vi "The Red LED.vi"() -> ()   [LabVIEW 2020]
uses:
  Red Button Enum.ctl
panel:
  out "error out":errorcluster
  in  "Open time duration(s)":u32=3
  in  "Switch":bool
  out "State":T1
  in  "stop":bool
  in  "1":bool
  in  "2":bool
  in  "3":bool
  out "Lamp":bool
  in  "Check for every step":bool
  # "The password is \"1-2-3\" consequtively, you should push \"check for every step\" in each step\nafter you select the number,  then switch and red LED indicator will be enabled. So as last step turn on the switch, LED will be open for 3 secs by default. You can easily change the password by giving desired boolean values inside case structure in the 1,2,3 cases, in the block diagram."
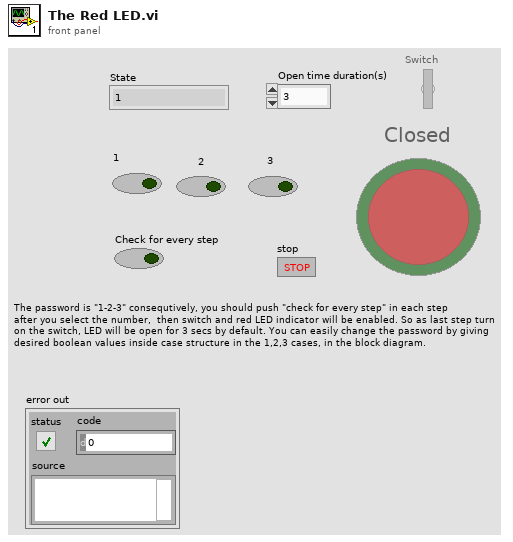
[diagram p1: front panel]
types:
  T1 = typedef "Red Button Enum.ctl" = enum16{"1", "2", "3", "Unlocked", "Open"}
  T2 = enum8{"Enabled", "Disabled", "Disabled and Grayed Out"}
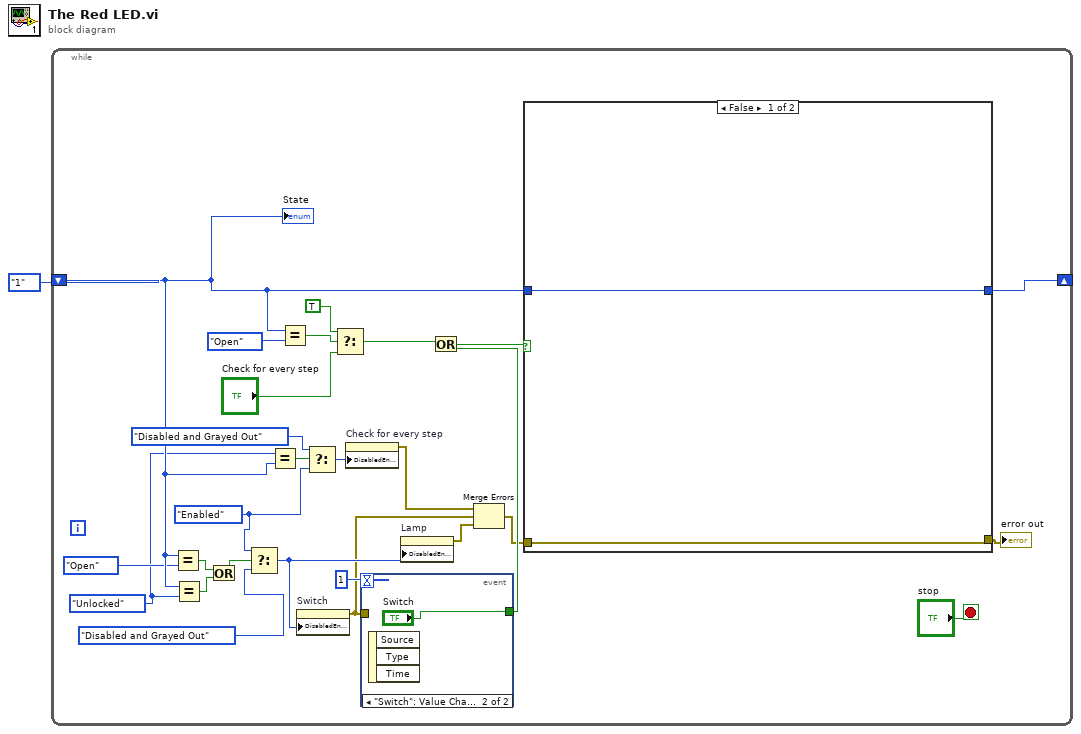
[diagram p0: block diagram]
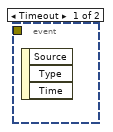
[diagram p2: hidden frame]
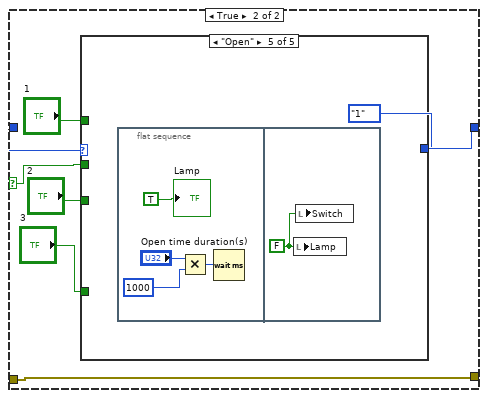
[diagram p3: hidden frame]
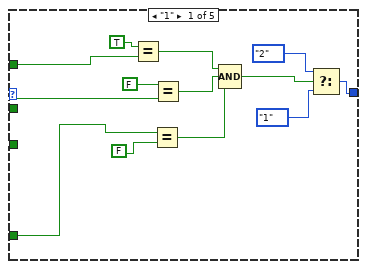
[diagram p4: hidden frame]
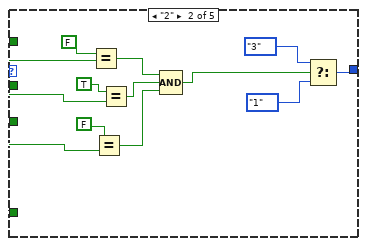
[diagram p5: hidden frame]
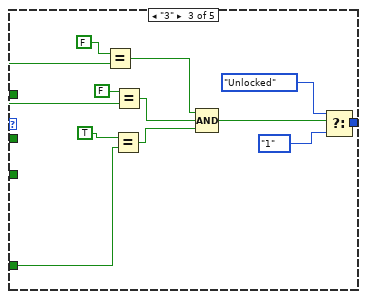
[diagram p6: hidden frame]
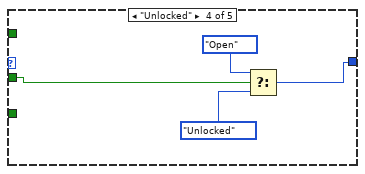
[diagram p7: hidden frame]
diagram:
  n1 = while {
    shift-right: [w27] -> _
    shift-left: Red_Button_Enum."1" ("Enum") -> [w13]
    stop <- "stop" stop-if-true
    w9 = T2."Enabled" ("Disabled")
    w7 = Red_Button_Enum."Unlocked" ("Enum")
    n2 = Equal?(x=w13, y=Red_Button_Enum."Open" ("Enum")) -> (x = y?=w21:bool)
    n3 = Equal?(x=w13, y=w7) -> (x = y?=w20:bool)
    n4 = Or(x=w21, y=w20) -> (x .or. y?=w19:bool)
    n5 = Select(t=w9, s=w19, f=T2."Disabled and Grayed Out" ("Disabled")) -> (s? t:f=w18:T2)
    n6 = Equal?(x=w7, y=w13) -> (x = y?=w11:bool)
    n7 = Equal?(x=w13, y=Red_Button_Enum."Open" ("Enum")) -> (x = y?=w26:bool)
    n8 = property on="Switch" class="Bool (strict)"("DisabledEnum"=w18) -> (error out=w4:errorcluster)  [unwired: 2 in, 1 out]
    n9 = Select(t=T2."Disabled and Grayed Out" ("Disabled"), s=w11, f=w9) -> (s? t:f=w8:T2)
    n10 = Select(t=TRUE, s=w26, f="Check for every step") -> (s? t:f=w16:bool)
    n11 = property on="Check for every step" class="Bool"("DisabledEnum"=w8) -> (error out=w5:errorcluster)  [unwired: 2 in, 1 out]
    n12 = event shown="[1] \"Switch\": Value Change" {
      selector: _ -> [_ _]
      dyn-events: _ -> [_ _]
      timeout: 1 -> [_ _]
      tunnel: w4 -> [_ _]
      tunnel: [_ "Switch"] -> w15
      event Timeout {
        n13 = event-data() -> ()  [unwired: 1 in, 3 out]
      }
      event "Switch": Value Change {
        n14 = event-data() -> ()  [unwired: 1 in, 3 out]
      }
    }
    n15 = property on="Lamp" class="Bool"("DisabledEnum"=w18) -> (error out=w3:errorcluster)  [unwired: 2 in, 1 out]
    n16 = Or(x=w16, y=w15) -> (x .or. y?=w14:bool)
    n17 = Merge Errors(w5, w4, w3) -> (w2:errorcluster)
    n18 = case shown="False" w14 {
      selector: w14 -> [_ w33]
      tunnel: w13 -> [w31 w34]
      tunnel: [w31 w38] -> w27
      tunnel: w2 -> [w30 w32]
      tunnel: [w30 w32] -> w6
      frame False {
      }
      frame True {
        n19 = case shown="\"Open\"" w34 {
          tunnel: [w44 w64 w77 w81 Red_Button_Enum."1" ("Enum")] -> w38
          tunnel: "1" -> [w43 w56 w69 _ _]
          tunnel: "2" -> [w42 w55 w68 _ _]
          tunnel: "3" -> [w41 w54 w67 _ _]
          tunnel: w33 -> [_ _ _ w78 _]
          frame "1" {
            n20 = Equal?(x=TRUE, y=w43) -> (x = y?=w48:bool)
            n21 = Equal?(x=w41, y=FALSE) -> (x = y?=w46:bool)
            n22 = Equal?(x=FALSE, y=w42) -> (x = y?=w47:bool)
            n23 = Compound Arithmetic op=AND(w48, w47, w46) -> (w45:bool)
            n24 = Select(t=Red_Button_Enum."2" ("Enum"), s=w45, f=Red_Button_Enum."1" ("Enum")) -> (s? t:f=w44:T1)
          }
          frame "2" {
            n25 = Equal?(x=FALSE, y=w56) -> (x = y?=w60:bool)
            n26 = Equal?(x=FALSE, y=w54) -> (x = y?=w58:bool)
            n27 = Equal?(x=TRUE, y=w55) -> (x = y?=w59:bool)
            n28 = Compound Arithmetic op=AND(w60, w59, w58) -> (w57:bool)
            n29 = Select(t=Red_Button_Enum."3" ("Enum"), s=w57, f=Red_Button_Enum."1" ("Enum")) -> (s? t:f=w64:T1)
          }
          frame "3" {
            n30 = Equal?(x=FALSE, y=w69) -> (x = y?=w73:bool)
            n31 = Equal?(x=TRUE, y=w67) -> (x = y?=w71:bool)
            n32 = Equal?(x=FALSE, y=w68) -> (x = y?=w72:bool)
            n33 = Compound Arithmetic op=AND(w73, w72, w71) -> (w70:bool)
            n34 = Select(t=Red_Button_Enum."Unlocked" ("Enum"), s=w70, f=Red_Button_Enum."1" ("Enum")) -> (s? t:f=w77:T1)
          }
          frame "Unlocked" {
            n35 = Select(t=Red_Button_Enum."Open" ("Enum"), s=w78, f=Red_Button_Enum."Unlocked" ("Enum")) -> (s? t:f=w81:T1)
          }
          frame "Open" {
            n36 = flat-sequence {
              frame #0 {
                n37 = Multiply(x="Open time duration(s)", y=u32 1000) -> (x*y=w83:u32)
                n38 = Wait (ms)(milliseconds to wait=w83) -> ()  [unwired: 1 out]
                "Lamp" <- TRUE ("Lamp")
              }
              frame #1 {
                w87 = FALSE ("Lamp")
                n39 = local write "Lamp"(w87) -> ()
                n40 = local write "Switch"(w87) -> ()
              }
            }
          }
        }
      }
    }
    "error out" <- w6
    "State" <- w13
  }
